vi "Has Destroyed.vi"(7 "Sender":refnum<class "Sender.lvclass">, 9 "Error":errorcluster, 10 "Actor":refnum<class "Actor.lvclass">, 11 "TEMPLATE Actor in":refnum<class "TEMPLATE Actor.lvclass">) -> (0 "Error out":errorcluster, 3 "TEMPLATE Actor out":refnum<class "TEMPLATE Actor.lvclass">)   [LabVIEW 2025]
uses:
  TEMPLATE Actor.lvclass
  <vilib>/Nathan Davis/jettl/jettl/jettl/Actor/Actor/Actor.lvclass
  <vilib>/Nathan Davis/jettl/jettl/jettl/Sender/Sender/Sender.lvclass
  TEMPLATE Actor.lvclass/TEMPLATE Actor.ctl
  C:/Users/nathan.davis/Desktop/dumb/TEMPLATE Actor/TEMPLATE Actor/TEMPLATE Actor.lvclass
  C:/Program Files/National Instruments/LabVIEW 2025/vi.lib/Nathan Davis/jettl/jettl/jettl/Actor/Actor/Actor.lvclass
  C:/Program Files/National Instruments/LabVIEW 2025/vi.lib/Nathan Davis/jettl/jettl/jettl/Has Destroyed Msg/Has Destroyed/Has Destroyed.lvclass
  C:/Users/nathan.davis/Desktop/dumb/Update Pump State Msg/Update Pump State/Update Pump State.lvclass
  <vilib>/Nathan Davis/jettl/jettl/jettl/Has Destroyed Msg/Has Destroyed Msg.lvlib
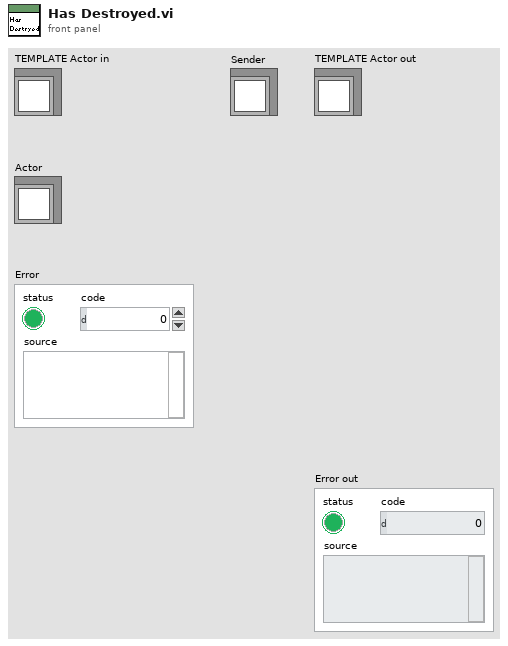
[diagram p1: front panel]
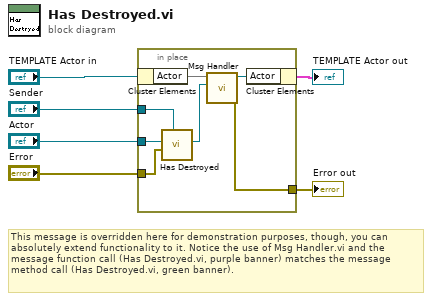
[diagram p0: block diagram]
diagram:
  # "This message is overridden here for demonstration purposes, though, you can absolutely extend functionality to it. Notice the use of Msg Handler.vi and the message function call (Has Destroyed.vi, purple banner) matches the message method call (Has Destroyed.vi, green banner)."
  n1 = in-place {
    in-place-border: [w11] -> w4
    in-place-border: "Sender" -> [w10]
    in-place-border: "Error" -> [w9]
    in-place-border: "Actor" -> [w8]
    n2 = in-place-cluster #1("TEMPLATE Actor in") -> ("Actor"=w13)
    n3 = call <vilib>:"Has Destroyed.vi"("Sender"=w10, "Error"=w9, "Actor"=w8) -> ("Msg"=w7:refnum<class "Msg.lvclass">)  [unwired: 8 in]
    n4 = call-dynamic "Msg Handler.vi"("Msg"=w7, "Actor in"=w13) -> ("Error out"=w11:errorcluster, "Actor out"=w12:refnum<class "Actor.lvclass">)  [unwired: 8 in]
    n5 = in-place-cluster #1("Actor"=w12) -> (→"TEMPLATE Actor out":cluster{})
  }
  "Error out" <- w4
